vi "3PhaseInverter.vi"() -> ()   [LabVIEW 2021]
uses:
  <vilib>/eio/EIONode/EIONode.xnode
  <vilib>/rvi/eio/common/nirviEmuTemplateMethod_errors.vi
panel:
  out "D05":bool
  out "D04":bool
  out "D03":bool
  out "D02":bool
  out "D01":bool
  out "D00":bool
  out "lut value at index":i16
  out "Index":i32
  out "Phase C":i16
  out "Phase A":i16
  out "Phase B":i16
  out "Current Time":u32
  out "Previous Time":u32
  out "Tick Count(Ticks)":u32
  out "needed pre conversion":fxp<+,32,16>
  in  "Frequency":i32
  out "ticks needed post conversion":fxp<+/-,64,34>
  in  "SET DESIRED TICK":u32
  in  "Math":bool
  in  "PUT DIFFERENCE":i32
  out "Saw tooth \nactual freq":fxp<+,32,16>
  in  "Sin":bool
  out "Difference Between":u32
  in  "main":bool
  # "HOW TO USE:\n1) set desired SIN frequency\n2) the outputted ticks needed will be provided \nto find a frequency for the sawtooth ath is minimum 15x greater!\n!!!\nIF YOU PUT A DESIRED TICK SMALLER THAN THE NEEDED IT WILL\nPROVIDE A HIGHER FREQUENCY , A LARGER WILL BE SMALLER\n!!!"
  # "This is to calculate the actual frequency, put inside the difference\nto see what our lookup tabe output is actualy being worked at"
  # "Where difference is derived"
  # "IGNORE FOR NOW!!! HAVENT IMPLEMENTED\nchecks comparison of carrier and sin"
  # "This just reads out \nvalues from sin wave"
  # "Checks index and LUT values"
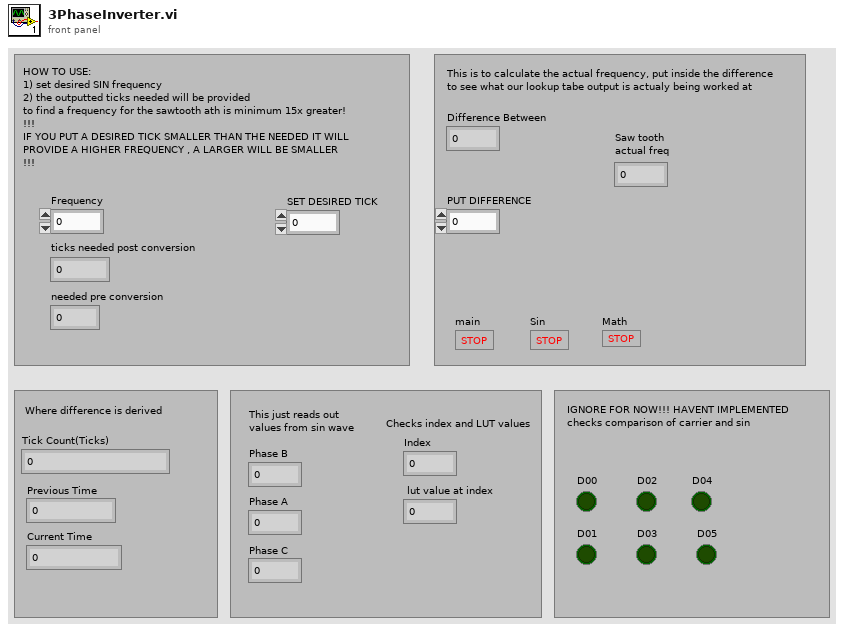
[diagram p1: front panel]
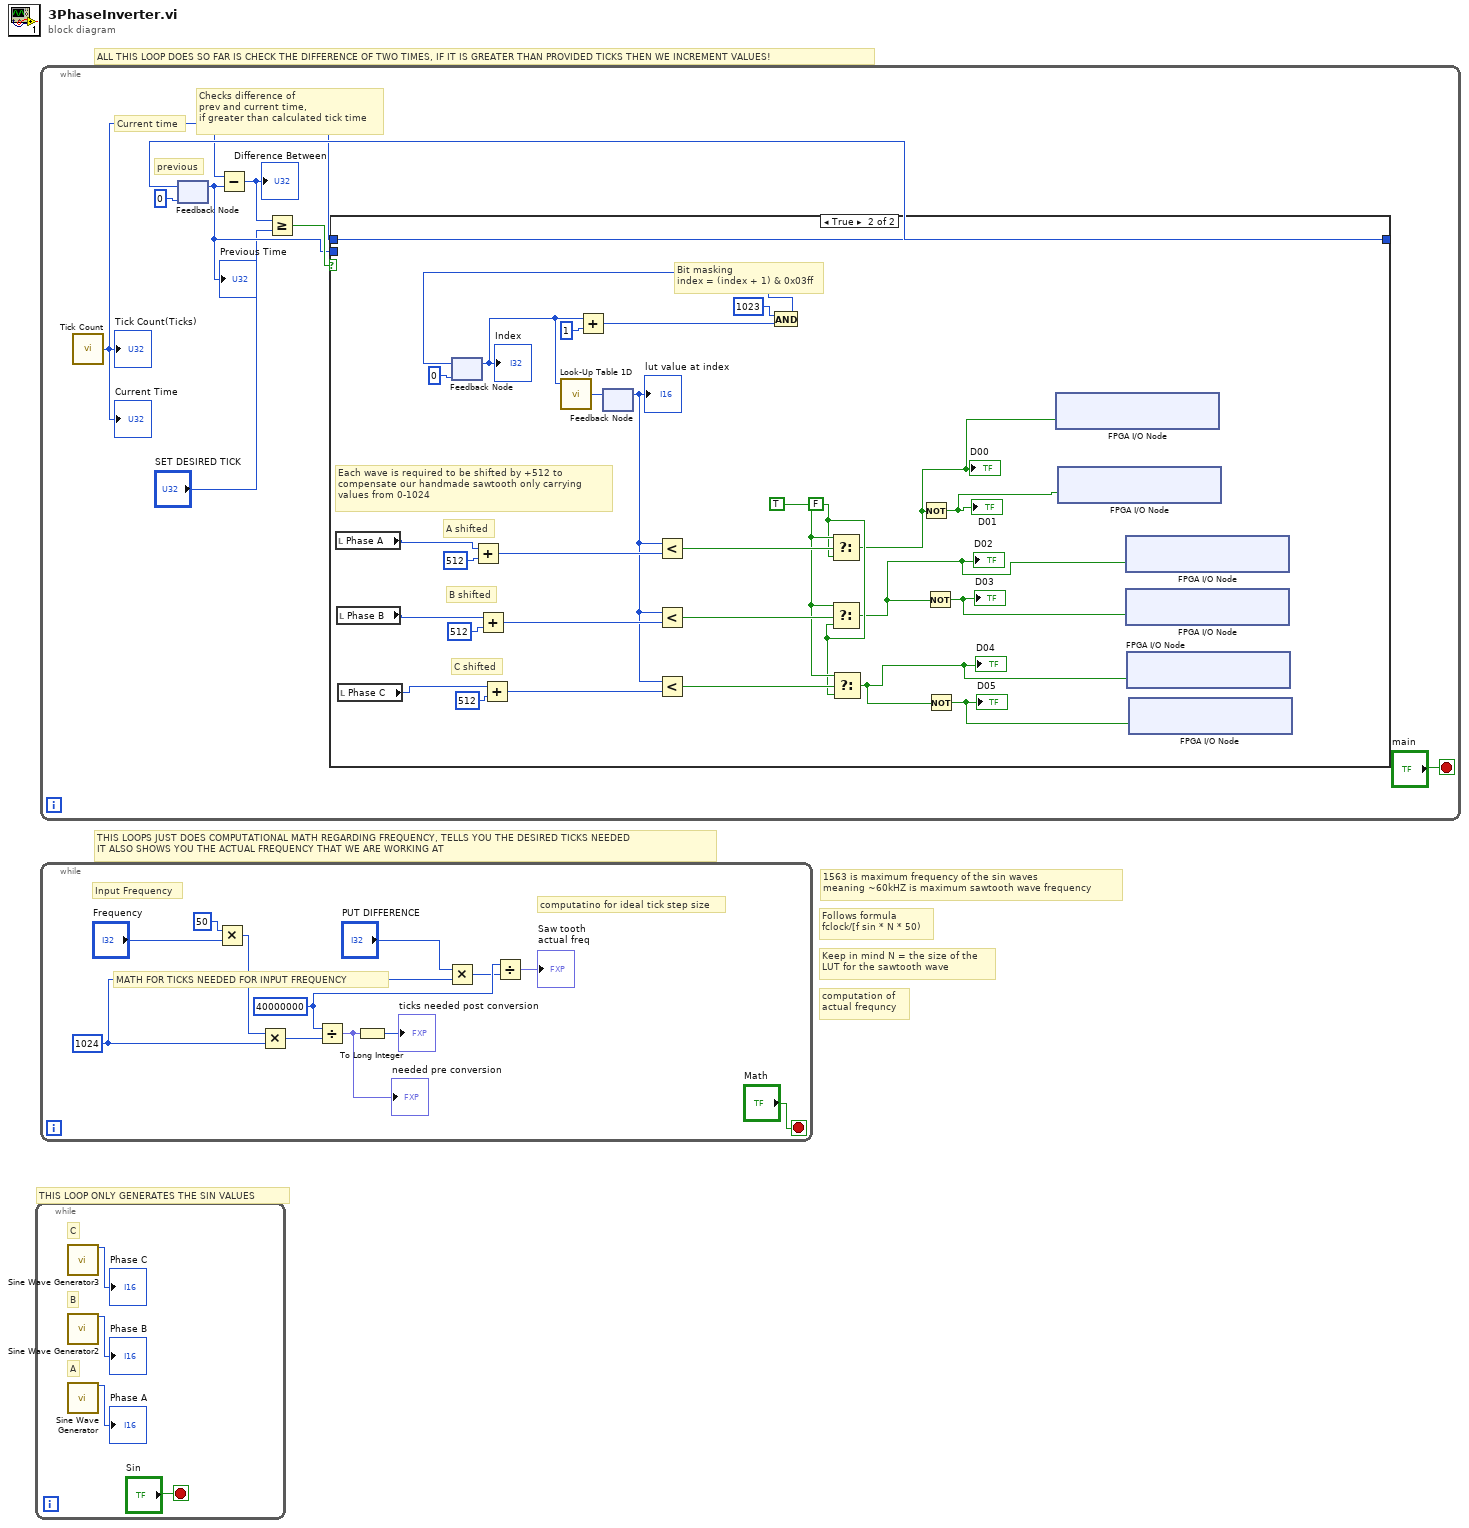
[diagram p0: block diagram]
diagram:
  # "ALL THIS LOOP DOES SO FAR IS CHECK THE DIFFERENCE OF TWO TIMES, IF IT IS GREATER THAN PROVIDED TICKS THEN WE INCREMENT VALUES!"
  # "computation of \nactual frequncy"
  # "1563 is maximum frequency of the sin waves \nmeaning ~60kHZ is maximum sawtooth wave frequency"
  # "Keep in mind N = the size of the \nLUT for the sawtooth wave"
  # "Follows formula \nfclock/[f sin * N * 50)"
  # "THIS LOOPS JUST DOES COMPUTATIONAL MATH REGARDING FREQUENCY, TELLS YOU THE DESIRED TICKS NEEDED\nIT ALSO SHOWS YOU THE ACTUAL FREQUENCY THAT WE ARE WORKING AT"
  # "THIS LOOP ONLY GENERATES THE SIN VALUES"
  n1 = while {
    stop <- "Sin" stop-if-true
    # "C"
    # "A"
    # "B"
    n2 = call "Sine Wave Generator3"() -> ("sine out"=→"Phase C":i16)  [unwired: 15 in]
    n3 = call "Sine Wave Generator2"() -> ("sine out"=→"Phase B":i16)  [unwired: 15 in]
    n4 = call "Sine Wave Generator"() -> ("sine out"=→"Phase A":i16)  [unwired: 15 in]
  }
  n5 = while {
    stop <- "main" stop-if-true
    # "Checks difference of \nprev and current time, \nif greater than calculated tick time"
    # "previous"
    # "Current time"
    n6 = call "Tick Count"() -> ("Tick Count(Ticks)"=w6:u32)
    "Tick Count(Ticks)" <- w6
    "Current Time" <- w6
    n7 = feedback #1(u32 0 ("Tick Count(Ticks)")) -> (w9:u32)
    "Previous Time" <- w9
    n8 = Subtract(x=w6, y=w9) -> (x-y=w7:u32)
    "Difference Between" <- w7
    n9 = Greater Or Equal?(x=w7, y="SET DESIRED TICK") -> (x >= y?=w11:bool)
    n10 = case shown="True" w11 {
      tunnel: w6 -> [_ w41]
      tunnel: [w13 w41] -> w10
      tunnel: w9 -> [w13 _]
      frame False {
      }
      frame True {
        w20 = FALSE
        w21 = TRUE
        # "Each wave is required to be shifted by +512 to \ncompensate our handmade sawtooth only carrying \nvalues from 0-1024"
        # "Bit masking \nindex = (index + 1) & 0x03ff"
        # "C shifted"
        # "B shifted"
        # "A shifted"
        n11 = local read "Phase A"() -> (w25:i16)
        n12 = local read "Phase B"() -> (w26:i16)
        n13 = local read "Phase C"() -> (w27:i16)
        n14 = feedback #2(i16 0) -> (w31:i16)
        "Index" <- w31
        n15 = Add(x=w25, y=u32 512) -> (x+y=w35:u32)
        n16 = Add(x=w26, y=u64 512) -> (x+y=w37:u64)
        n17 = Add(x=w27, y=u32 512) -> (x+y=w36:u32)
        n18 = call "Look-Up Table 1D"("address"=w31) -> ("data out"=w34:i16)  [unwired: 8 in]
        n19 = Add(x=w31, y=i16 1) -> (x+y=w30:i16)
        n20 = feedback #3() -> (w33:i16)  [unwired: 1 in]
        "lut value at index" <- w33
        n21 = feedback-in #3(w34) -> ()
        n22 = Less?(x=w33, y=w35) -> (x < y?=w22:bool)
        n23 = Less?(x=w33, y=w37) -> (x < y?=w23:bool)
        n24 = Less?(x=w33, y=w36) -> (x < y?=w24:bool)
        n25 = And(x=i16 1023, y=w30) -> (x .and. y?=w28:i16)
        n26 = feedback-in #2(w28) -> ()
        n27 = Select(t=w21, s=w22, f=w20) -> (s? t:f=w19:bool)
        "D00" <- w19
        n28 = Select(t=w21, s=w23, f=w20) -> (s? t:f=w17:bool)
        "D02" <- w17
        n29 = Select(t=w21, s=w24, f=w20) -> (s? t:f=w14:bool)
        "D04" <- w14
        n30 = Not(x=w19) -> (.not. x?=w18:bool)
        "D01" <- w18
        n31 = Not(x=w17) -> (.not. x?=w16:bool)
        "D03" <- w16
        n32 = Not(x=w14) -> (.not. x?=w15:bool)
        "D05" <- w15
        n33 = xnode "FPGA I/O Node"("RMC/Half-Bridge/DO0"=w19) -> ()  [unwired: 1 in, 1 out]
        n34 = xnode "FPGA I/O Node"("RMC/Half-Bridge/DO1"=w18) -> ()  [unwired: 1 in, 1 out]
        n35 = xnode "FPGA I/O Node"("RMC/Half-Bridge/DO2"=w17) -> ()  [unwired: 1 in, 1 out]
        n36 = xnode "FPGA I/O Node"("RMC/Half-Bridge/DO3"=w16) -> ()  [unwired: 1 in, 1 out]
        n37 = xnode "FPGA I/O Node"("RMC/Half-Bridge/DO4"=w14) -> ()  [unwired: 1 in, 1 out]
        n38 = xnode "FPGA I/O Node"("RMC/Half-Bridge/DO5"=w15) -> ()  [unwired: 1 in, 1 out]
      }
    }
    n39 = feedback-in #1(w10) -> ()
  }
  n40 = while {
    stop <- "Math" stop-if-true
    w48 = 1024
    w49 = 40000000
    # "MATH FOR TICKS NEEDED FOR INPUT FREQUENCY"
    # "computatino for ideal tick step size"
    # "Input Frequency"
    n41 = Multiply(x=50, y="Frequency") -> (x*y=w53:i32)
    n42 = Multiply(x=w53, y=w48) -> (x*y=w52:i32)
    n43 = Divide(x=w49, y=w52) -> (x/y=w51:fxp<+,32,16>)
    "needed pre conversion" <- w51
    n44 = To Long Integer(number=w51) -> (32bit integer=→"ticks needed post conversion":i32)
    n45 = Multiply(x="PUT DIFFERENCE", y=w48) -> (x*y=w47:u32)
    n46 = Divide(x=w49, y=w47) -> (x/y=→"Saw tooth \nactual freq":fxp<+,32,16>)
  }
